vi "Configure Math (FFT).vi"(7 "FFT Scale (0: DBV)":u16(ring) items=["dBV", "Linear"], 8 "error in (no error)":errorcluster, 9 "FFT Window (0: Hanning)":u16(ring) items=["Hanning", "Rectangular", "Hamming", "Blackman-Harris"], 10 "FFT Source (0: Channel 1)":u16(ring) items=["Channel 1"=0, "Channel 2"=1, "Channel 3"=2, "Channel 4"=3, "Reference 1"=5, "Reference 2"=6, "Reference 3"=7, "Reference 4"=8], 11 "VISA resource name":refnum<visa-resource-name>) -> (0 "error out":errorcluster, 3 "VISA resource name out":refnum<visa-resource-name>)   [LabVIEW 2016, in "Tektronix DPO MSO 2000 4000 Series.lvlib"]
doc: "Configures a math channel to calculate an FFT."
uses:
  Tektronix DPO MSO 2000 4000 Series.lvlib
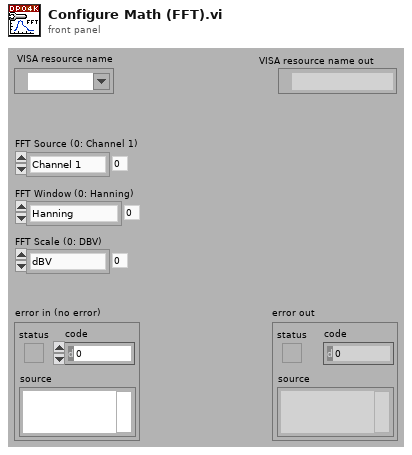
[diagram p1: front panel]
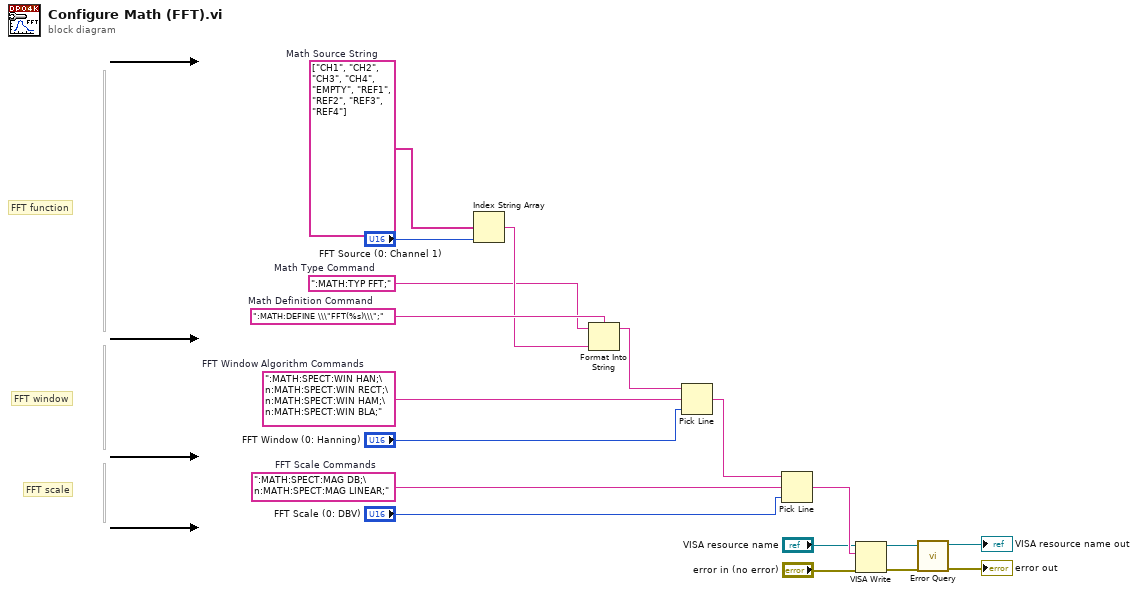
[diagram p0: block diagram]
diagram:
  w3 = string[] ["CH1", "CH2", "CH3", "CH4", "EMPTY", "REF1", "REF2", "REF3", "REF4"]  # Math Source String
  w4 = ":MATH:TYP FFT;"  # Math Type Command
  w14 = ":MATH:SPECT:WIN HAN;\n:MATH:SPECT:WIN RECT;\n:MATH:SPECT:WIN HAM;\n:MATH:SPECT:WIN BLA;"  # FFT Window Algorithm Commands
  w15 = ":MATH:SPECT:MAG DB;\n:MATH:SPECT:MAG LINEAR;"  # FFT Scale Commands
  w17 = ":MATH:DEFINE \\\"FFT(%s)\\\";"  # Math Definition Command
  # "FFT scale"
  # "FFT window"
  # "FFT function"
  n1 = Index String Array(1:"FFT Source (0: Channel 1)", 2:w3) -> (0:w16:string)  [unwired: 1 in]
  n2 = Format Into String(format string=w17, initial string=w4, w16) -> (resulting string=w12:string)  [unwired: 1 in, 1 out]
  n3 = Pick Line(string ("")=w12, multi-line string=w14, line index="FFT Window (0: Hanning)") -> (output string=w10:string)
  n4 = Pick Line(string ("")=w10, multi-line string=w15, line index="FFT Scale (0: DBV)") -> (output string=w5:string)
  n5 = VISA Write(VISA resource name="VISA resource name", write buffer=w5, error in (no error)="error in (no error)") -> (VISA resource name out=w9:refnum<visa-resource-name>, error out=w8:errorcluster)  [unwired: 1 out]
  n6 = call "Error Query.vi"("error in (no error)"=w8, "VISA resource name"=w9) -> ("error out"=→"error out":errorcluster, "VISA resource name out"=→"VISA resource name out":refnum<visa-resource-name>)  [unwired: 6 in, 2 out]
